vi "Date-Time string to DT format.vi"(1 "date/time string":string) -> (0 "Resulting Time Stamp":timestamp)   [LabVIEW 2010]
doc: "This VI convert a date/time string back to a time stamp."
uses:
  <vilib>/Utility/miscctls.llb/LVDateTimeRec.ctl
panel:
  out "Numeric":i32
  # "This control should have data in the form:\n4/30/2004 7:48:47 PM"
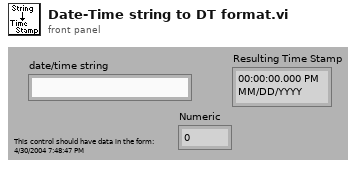
[diagram p1: front panel]
types:
  T1 = typedef "LVDateTimeRec.ctl" = cluster{"fractional second":dbl, "second":i32, "minute":i32, "hour":i32, "day of month":i32, "month":i32, "year":i32, "day of week":i32, "day of year":i32, "DST":i32}
  T2 = cluster{"second":i32, "minute":i32, "hour":i32, "day of month":i32, "month":i32, "year":i32, "day of week":i32, "day of year":i32, "is DST":i32}
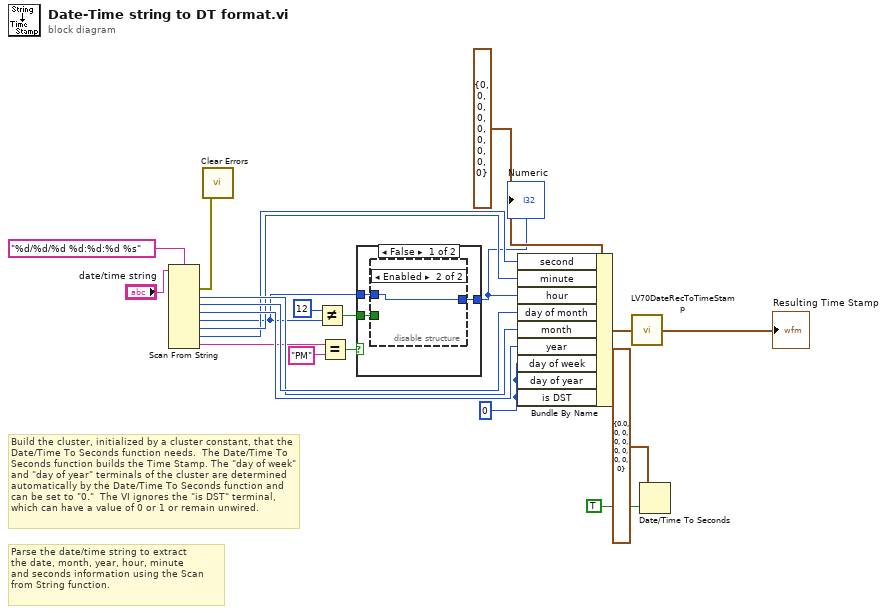
[diagram p0: block diagram]
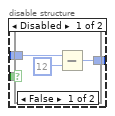
[diagram p2: hidden frame]
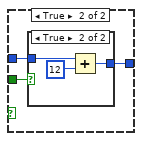
[diagram p4: hidden frame]
diagram:
  w17 = 0
  # "Build the cluster, initialized by a cluster constant, that the Date/Time To Seconds function needs.  The Date/Time To Seconds function builds the Time Stamp. The \"day of week\" and \"day of year\" terminals of the cluster are determined automatically by the Date/Time To Seconds function and can be set to \"0.\"  The VI ignores the \"is DST\" terminal, which can have a value of 0 or 1 or remain unwired."
  # "Parse the date/time string to extract \nthe date, month, year, hour, minute \nand seconds information using the Scan\nfrom String function."
  n1 = Scan From String "Scan From String"(format string="%d/%d/%d %d:%d:%d %s", input string="date/time string") -> (error out=w4:errorcluster, output 1=w15:i32, output 2=w16:i32, output 3=w14:i32, output 4=w8:i32, output 5=w13:i32, output 6=w12:i32, output 7=w11:string)  [unwired: 9 in, 2 out]
  n2 = call <vilib>:"Clear Errors.vi"("error in (no error)"=w4) -> ()  [unwired: 6 in, 1 out]
  n3 = Not Equal?(x=12 ("y"), y=w8) -> (x != y?=w5:bool)
  n4 = Equal?(x=w11, y="PM") -> (x = y?=w6:bool)
  n5 = case shown="False" w6 {
    tunnel: w8 -> [w24 w34]
    tunnel: [w22 w33] -> w7
    tunnel: w5 -> [w23 w35]
    frame False {
      n6 = disable-structure shown="Enabled" {
        disable-tunnel: w24 -> [w27 w32]
        disable-tunnel: w23 -> [w26 _]
        disable-tunnel: [w25 w32] -> w22
        frame Disabled {
          n7 = case shown="False" w26 {
            tunnel: w27 -> [w30 w31]
            tunnel: [w28 w31] -> w25
            frame False {
              n8 = Subtract(x=w30, y=12) -> (x-y=w28:i32)
            }
            frame True {
            }
          }
        }
        frame Enabled {
        }
      }
    }
    frame True {
      n9 = case shown="True" w35 {
        tunnel: w34 -> [w36 w38]
        tunnel: [w36 w37] -> w33
        frame False {
        }
        frame True {
          n10 = Add(x=w38, y=12) -> (x+y=w37:i32)
        }
      }
    }
  }
  "Numeric" <- w7
  n11 = Bundle By Name(cluster=T2 {"second"=0, "minute"=0, "hour"=0, "day of month"=0, "month"=0, "year"=0, "day of week"=0, "day of year"=0, "is DST"=0} ("date time rec"), "second"=w12, "minute"=w13, "hour"=w7, "day of month"=w16, "month"=w15, "year"=w14, "day of week"=w17, "day of year"=w17, "is DST"=w17) -> (w3:T2)
  n12 = call <vilib>:"LV70DateRecToTimeStamp.vi"("date time rec"=w3) -> ("Time Stamp"=→"Resulting Time Stamp":timestamp)
  n13 = Date/Time To Seconds(1:TRUE ("is UTC (F)"), 2:T1 {"fractional second"=0.0, "second"=0, "minute"=0, "hour"=0, "day of month"=0, "month"=0, "year"=0, "day of week"=0, "day of year"=0, "DST"=0} ("date time rec")) -> ()  [unwired: 1 out]
